vi "time.vi"(6 "timeout (25000ms)":i32=25000, 8 "error in (no error)":errorcluster, 11 "daemon reference in":refnum<k5>) -> (0 "error out":errorcluster, 2 "target time":timestamp, 3 "daemon reference out":refnum<k5>, 5 "command out":string="time")   [LabVIEW 2017]
doc: "<b>Command: </b>\"time\"\n\n<b>Description: </b> Queries the target for the current time in the format \"DD/MM/YYYY HH:MM:SS\".\n\n<b>Parameters: </b> None\n____________________________________________\nDIPC 692 Daemon API 10.0.0.1\nSam Tee - Dyson Technology Ltd\nCopyright (c) 2024, Dyson Technology Ltd"
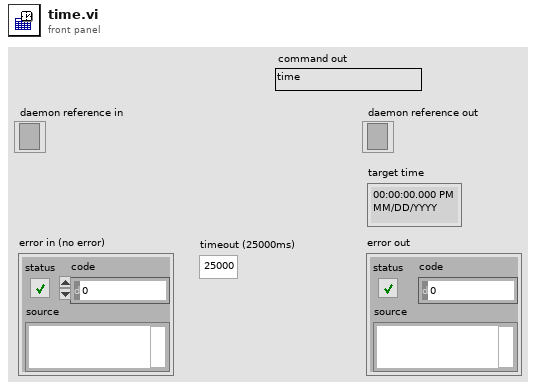
[diagram p1: front panel]
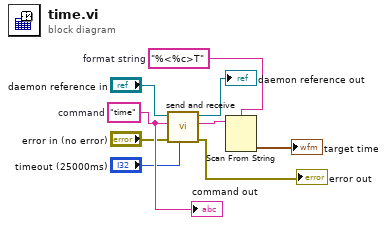
[diagram p0: block diagram]
diagram:
  w3 = "%<%c>T"  # format string
  w7 = "time"  # command
  n1 = call "send and receive.vi"("timeout (25000ms)"="timeout (25000ms)", "error in (no error)"="error in (no error)", "command"=w7, "daemon reference in"="daemon reference in") -> ("error out"=→"error out":errorcluster, "response"=w4:string, "daemon reference out"=→"daemon reference out":refnum<k5>)  [unwired: 5 in]
  n2 = Scan From String(format string=w3, input string=w4) -> (output 1=→"target time":timestamp)  [unwired: 3 in, 3 out]
  "command out" <- w7
